vi "Mexa read U.vi"() -> (2 "Output":u8[](array[numeric]))   [LabVIEW 2014]
uses:
  <vilib>/rvi/eio/common/nirviEmuTemplateMethod_errors.vi
  <vilib>/eio/EIOMethodNode/EIOMethodNode.xnode
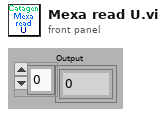
[diagram p1: front panel]
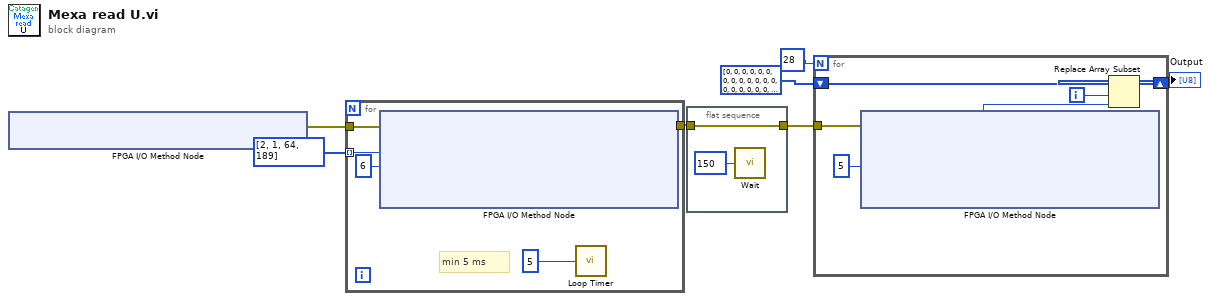
[diagram p0: block diagram]
diagram:
  n1 = xnode "FPGA I/O Method Node"() -> ("error out"=w3:errorcluster)  [unwired: 2 in, 1 out]
  n2 = for {
    tunnel: [w11] -> w2
    tunnel: u8[] [2, 1, 64, 189] -> [w10] mode=indexing
    tunnel: w3 -> [w8]
    # "min 5 ms"
    n3 = xnode "FPGA I/O Method Node"("error in"=w8, "Data"=w10, "Timeout (ms)"=6) -> ("error out"=w11:errorcluster)  [unwired: 1 in, 2 out]
    n4 = call "Loop Timer"("Count(mSec)"=u32 5 ("Count(mSec) 2")) -> ()  [unwired: 1 out]
  }
  n5 = flat-sequence {
    tunnel: w2 -> [w14]
    tunnel: [w14] -> w1
    frame #0 {
      n6 = call "Wait"("Count(mSec)"=u32 150) -> ()  [unwired: 1 out]
    }
  }
  n7 = for {
    N: 28 -> [_]
    tunnel: w1 -> [w20]
    shift-right: [w15] -> w4
    shift-left: u8[] [0, 0, 0, 0, 0, 0, 0, 0, 0, 0, 0, 0, 0, 0, 0, 0, 0, 0, 0, 0, 0, 0, 0, 0, 0, 0, 0, 0] -> [w18]
    i -> [w16]
    n8 = xnode "FPGA I/O Method Node"("error in"=w20, "Timeout (ms)"=5) -> ("Data"=w17:u8)  [unwired: 1 in, 3 out]
    n9 = Replace Array Subset(array=w18, new element=w17, index=w16) -> (w15:u8[])
  }
  "Output" <- w4
